vi "Utility Write Config INI to File.vi"(7 "File Type":string(combo)=".ini", 8 "Error In":errorcluster, 10 "reference":refnum<vi>, 11 "Path In":path) -> (0 "Error Out":errorcluster, 3 "Path Out":path)   [LabVIEW 2015]
uses:
  <vilib>/Utility/config.llb/Write Key (String).vi
  <vilib>/Utility/config.llb/NI_LVConfig.lvlib
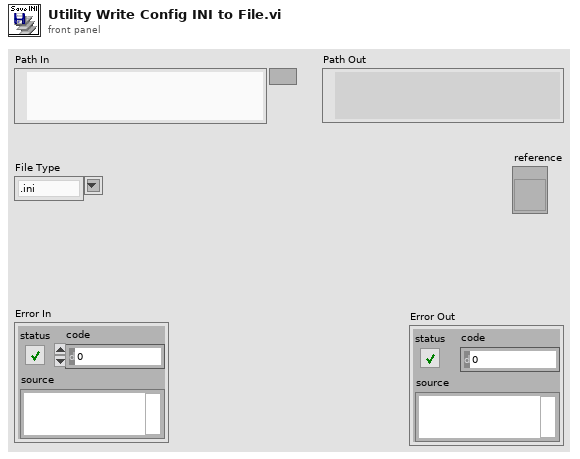
[diagram p1: front panel]
types:
  T1 = typedef "NI_LVConfig.lvlib/Config Data RefNum.ctl" = refnum<k1>
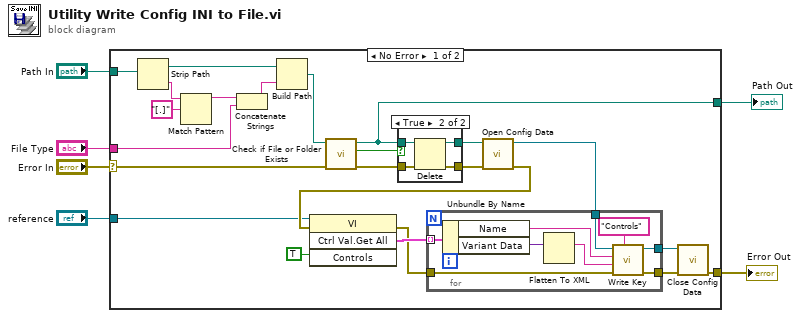
[diagram p0: block diagram]
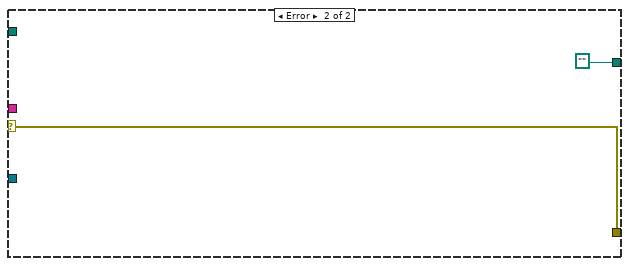
[diagram p3: hidden frame]
diagram:
  n1 = case shown="No Error" "Error In" {
    selector: "Error In" -> [w18 w46]
    tunnel: [w11 w46] -> w1
    tunnel: [w9 path ""] -> w6
    tunnel: "Path In" -> [w10 _]
    tunnel: "File Type" -> [w8 _]
    tunnel: "reference" -> [w7 _]
    frame No Error {
      n2 = Strip Path(path=w10) -> (stripped path=w28:path, name=w25:string)
      n3 = Match Pattern(string=w25, regular expression="[.]" ("search string")) -> (before substring=w26:string)  [unwired: 1 in, 3 out]
      n4 = Concatenate Strings(w26, w8) -> (w24:string)
      n5 = Build Path(base path=w28, name or relative path=w24) -> (appended path=w19:path)
      n6 = call <vilib>:"Check if File or Folder Exists.vi"("error in (no error)"=w18, "path"=w19) -> ("error out"=w22:errorcluster, "file or folder exists?"=w23:bool, "dup path"=w9:path)  [unwired: 7 in]
      n7 = case shown="True" w23 {
        tunnel: w22 -> [w39 w44]
        tunnel: w9 -> [w40 w43]
        tunnel: [w40 w42] -> w21
        tunnel: [w39 w41] -> w20
        frame False {
        }
        frame True {
          n8 = Delete(path (use dialog)=w43, error in=w44) -> (deleted path=w42:path, error out=w41:errorcluster)  [unwired: 3 in, 1 out]
        }
      }
      n9 = call <vilib>:"Open Config Data.vi"("error in (no error)"=w20, "configuration file path"=w21) -> ("error out"=w15:errorcluster, "refnum"=w16:T1)  [unwired: 1 in, 7 out]
      n10 = invoke class="VI" method="Ctrl Val.Get All"(reference=w7, error in=w15, "Controls"=TRUE) -> (error out=w14:errorcluster, "Get All Control Values Variant"=w17:cluster{"Name":string, "Variant Data":variant}[])  [unwired: 1 in, 2 out]
      n11 = for {
        tunnel: w17 -> [w38] mode=indexing
        tunnel: w16 -> [w35]
        tunnel: w14 -> [w34]
        tunnel: [w31] -> w13
        tunnel: [w30] -> w12
        n12 = Unbundle By Name(w38) -> ("Name"=w33:string, "Variant Data"=w37:variant)
        n13 = Flatten To XML(anything=w37) -> (xml string=w32:string)
        n14 = call-poly <vilib>:"Write Key.vi"("section"="Controls", "error in (no error)"=w34, "value"=w32, "key"=w33, "refnum"=w35) -> ("error out"=w30:errorcluster, "refnum out"=w31:T1)  [unwired: 4 in, 1 out]
      }
      n15 = call <vilib>:"Close Config Data.vi"("error in (no error)"=w12, "refnum"=w13) -> ("error out"=w11:errorcluster)  [unwired: 1 in, 8 out]
    }
    frame Error {
      (unwired) ""
    }
  }
  "Path Out" <- w6
  "Error Out" <- w1
